vi "de-queue for data stream.vi"(11 "Queues":T1) -> (0 "data":variant, 2 "message":string, 3 "Queues out":T1)   [LabVIEW 2018]
uses:
  type defs/Queues.ctl
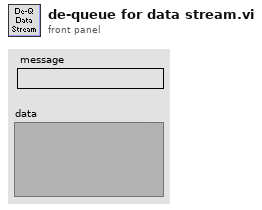
[diagram p1: front panel]
types:
  T1 = typedef "Queues.ctl" = cluster{"messageHandler":refnum<queue>, "comms":refnum<queue>, "dataStream":refnum<queue>, "dataProcessor":refnum<queue>, "fileIO":refnum<queue>, "userInterface":refnum<queue>, "errors":refnum<queue>, "customCompressor":refnum<queue>}
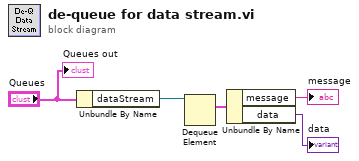
[diagram p0: block diagram]
diagram:
  n1 = Unbundle By Name("Queues") -> ("dataStream"=w4:refnum<queue>)
  n2 = Dequeue Element(queue=w4) -> (element=w3:cluster{"message":string, "data":variant})  [unwired: 2 in, 3 out]
  n3 = Unbundle By Name(w3) -> ("message"=→"message":string, "data"=→"data":variant)
  "Queues out" <- "Queues"
